vi "Set Class Instance.vi"(11 "OsciloscopeType":string) -> (3 "Obtain Class":refnum<class "OsciloscopeClass.lvclass">)   [LabVIEW 2020, in "Osciloscope Tektronix.lvlib"]
uses:
  Osciloscope Tektronix.lvlib
  Downloads/Osciloscope_AguayoSalma-develop/Osciloscope_AguayoSalma-develop/osiloscopio/Osciloscope/Class/Implementaciones/OsciloscopeClass/OsciloscopeClass.lvclass
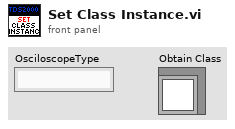
[diagram p1: front panel]
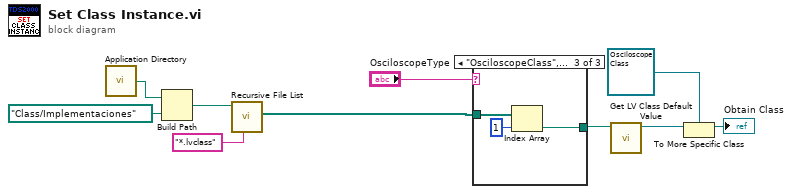
[diagram p0: block diagram]
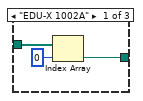
[diagram p2: hidden frame]
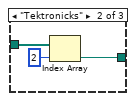
[diagram p3: hidden frame]
diagram:
  n1 = call <vilib>:"Application Directory.vi"() -> ("Application Directory"=w10:path)
  n2 = Build Path(base path=w10, name or relative path=path "Class/Implementaciones") -> (appended path=w8:path)
  n3 = call <vilib>:"Recursive File List.vi"("pattern"="*.lvclass", "Folder Path"=w8) -> ("All Files in Dir"=w5:path[])  [unwired: 5 in, 4 out]
  n4 = case shown="\"OsciloscopeClass\", Default" "OsciloscopeType" {
    tunnel: w5 -> [w13 w16 w19]
    tunnel: [w11 w14 w17] -> w4
    frame "EDU-X 1002A" {
      n5 = Index Array(array=w13, index=0) -> (element=w11:path)
    }
    frame "Tektronicks" {
      n6 = Index Array(array=w16, index=2) -> (element=w14:path)
    }
    frame "OsciloscopeClass", Default {
      n7 = Index Array(array=w19, index=1) -> (element=w17:path)
    }
  }
  n8 = call <vilib>:"Get LV Class Default Value.vi"("class path"=w4) -> ("object"=w3:refnum<class>)  [unwired: 9 in, 1 out]
  n9 = To More Specific Class(target class=refnum<class "OsciloscopeClass.lvclass"> refnum ("OsciloscopeClass.lvclass"), reference=w3) -> (specific class reference=→"Obtain Class":refnum<class "OsciloscopeClass.lvclass">)  [unwired: 1 in, 1 out]
